vi "sub_GSlam_fill-Hnb.vi"(9 "edge in":T2, 10 "b":T1, 11 "H":T1 caption="H in") -> (2 "b out":T1 caption="b", 3 "H out":T1)   [LabVIEW 2019]
uses:
  <vilib>/Analysis/Matrix/Datatypes/RealMatrix.ctl
  Ctrl/cmd_common.ctl
  <vilib>/Analysis/Matrix/Numeric/Multiply/Multiply - RM,RM.vi
  <vilib>/Analysis/Matrix/Numeric/Add/Add - RM,RM.vi
  <vilib>/Analysis/Matrix/NI_Matrix.lvlib
panel:
  out "H matrix":dbl[][](graph)
  out "열의 개수":i32
  out "행의 개수":i32
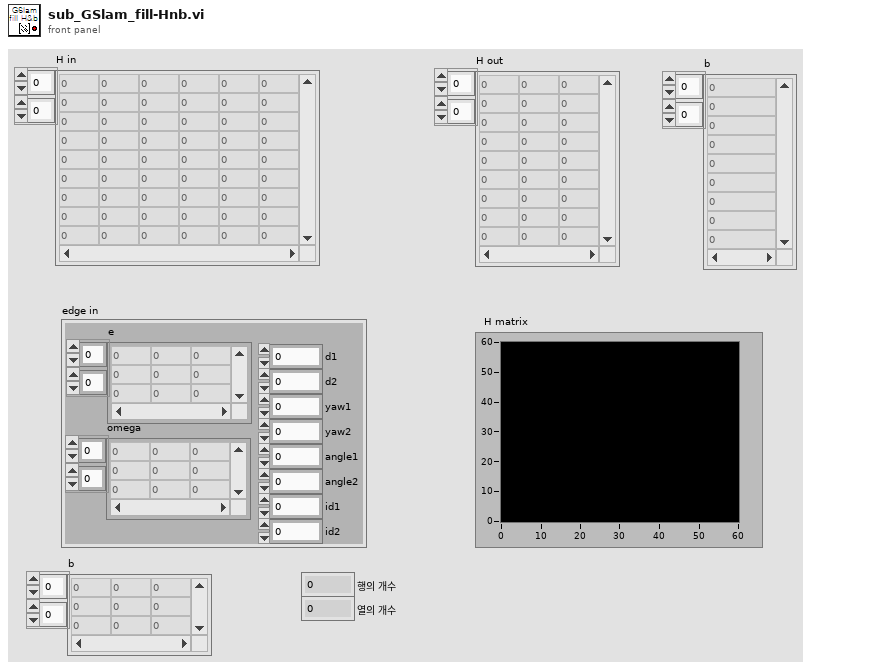
[diagram p1: front panel]
types:
  T1 = typedef "NI_Matrix.lvlib/RealMatrix.ctl" = dbl[][]
  T2 = cluster{"e":T1, "omega":T1, "d1":dbl, "d2":dbl, "yaw1":dbl, "yaw2":dbl, "angle1":dbl, "angle2":dbl, "id1":i32, "id2":i32}
  T3 = typedef "cmd_common.ctl" = enum16{"read", "write"}
  T4 = cluster{"Q Sim":T1, "R Sim":T1, "DT":dbl, "SIM_TIME":dbl, "MAX_RANGE":dbl, "STATE_SIZE":i32, "C_SIGMA 1":dbl, "C_SIGMA 2":dbl, "C_SIGMA 3":dbl, "MAX_ITR":u32}
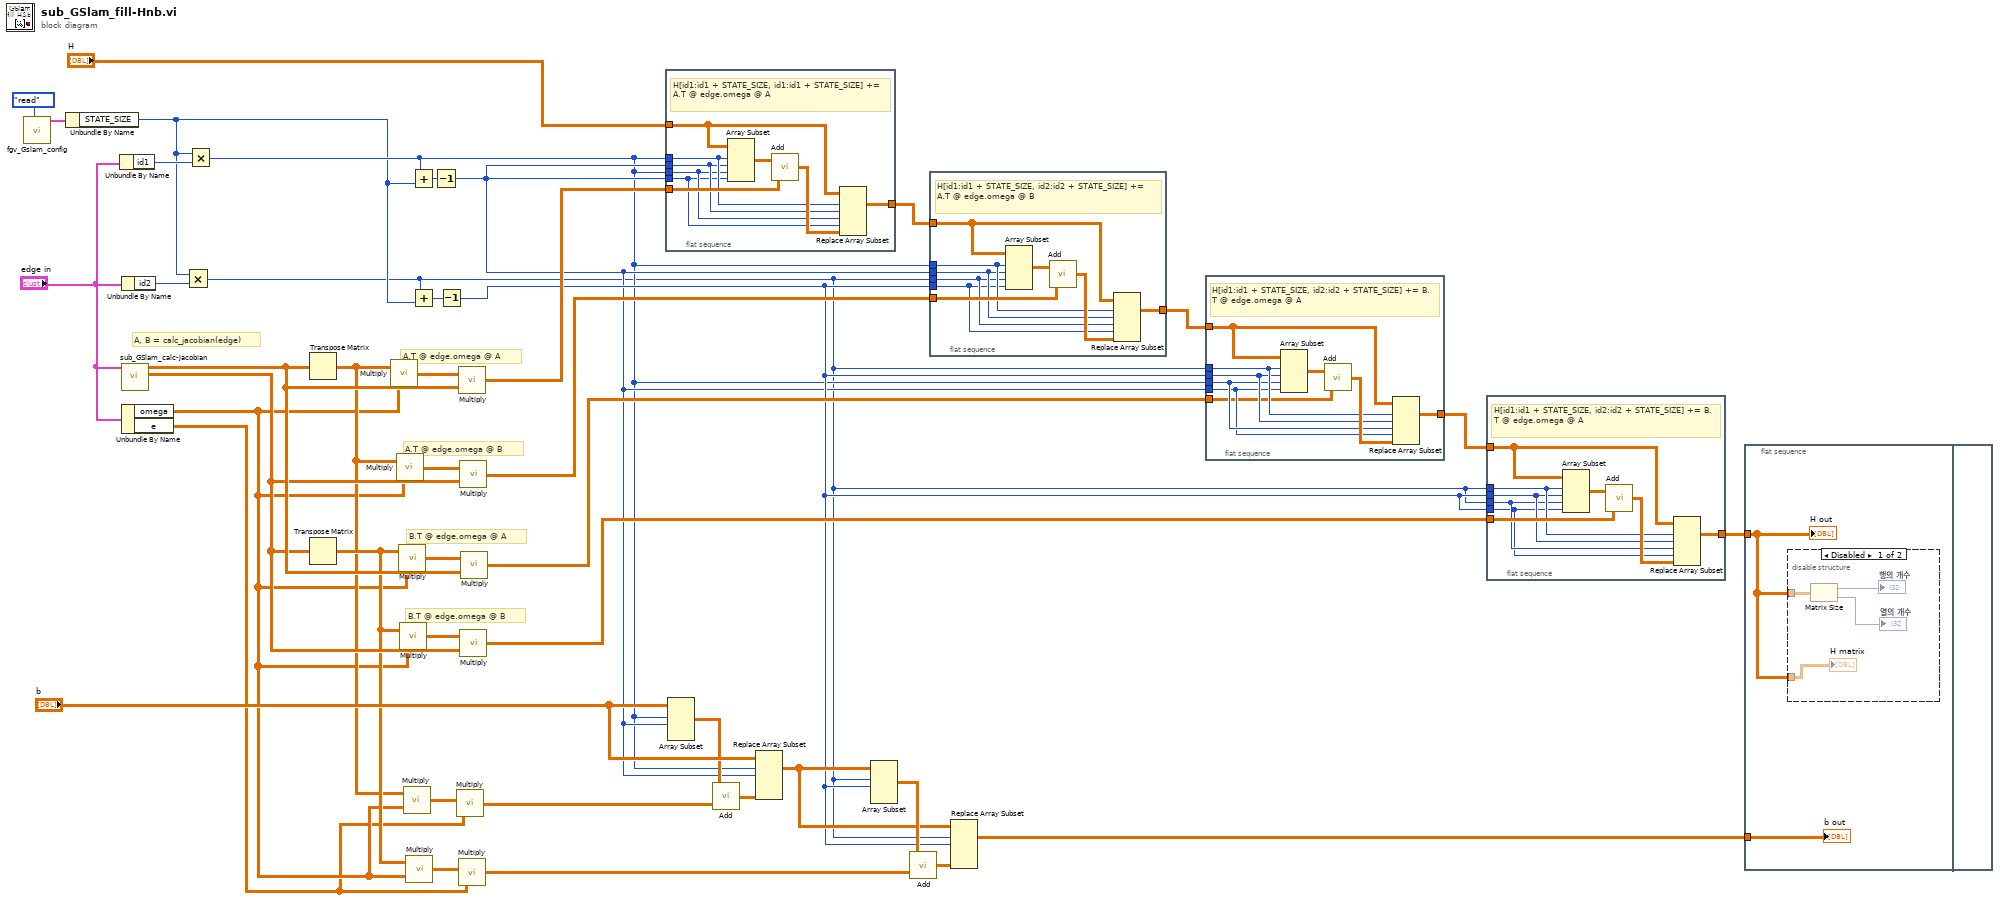
[diagram p0: block diagram]
diagram:
  # "B.T @ edge.omega @ B"
  # "B.T @ edge.omega @ A"
  # "A.T @ edge.omega @ B"
  # "A, B = calc_jacobian(edge)"
  # "A.T @ edge.omega @ A"
  n1 = call "fgv_Gslam_config.vi"("cmd"=cmd_common."read") -> ("G cofnig out"=w41:T4)  [unwired: 10 in]
  n2 = Unbundle By Name(w41) -> ("STATE_SIZE"=w6:i32)
  n3 = Unbundle By Name("edge in") -> ("id1"=w9:i32)
  n4 = Unbundle By Name("edge in") -> ("id2"=w7:i32)
  n5 = call "sub_GSlam_calc-jacobian.vi"("edge"="edge in") -> ("B"=w32:T1, "A"=w33:T1)  [unwired: 9 in]
  n6 = Unbundle By Name("edge in") -> ("omega"=w3:T1, "e"=w2:T1)
  n7 = Multiply(x=w6, y=w7) -> (x*y=w5:i32)
  n8 = Multiply(x=w6, y=w9) -> (x*y=w8:i32)
  n9 = Transpose Matrix(1:w33) -> (0:w4:T1)
  n10 = Transpose Matrix(1:w32) -> (0:w18:T1)
  n11 = call-poly <vilib>:"Multiply.vi"("Real Matrix B"=w3, "Real Matrix A"=w4) -> ("A * B"=w40:T1)
  n12 = call-poly <vilib>:"Multiply.vi"("Real Matrix B"=w3, "Real Matrix A"=w4) -> ("A * B"=w37:T1)
  n13 = call-poly <vilib>:"Multiply.vi"("Real Matrix B"=w3, "Real Matrix A"=w18) -> ("A * B"=w35:T1)
  n14 = call-poly <vilib>:"Multiply.vi"("Real Matrix B"=w3, "Real Matrix A"=w18) -> ("A * B"=w34:T1)
  n15 = call-poly <vilib>:"Multiply.vi"("Real Matrix B"=w3, "Real Matrix A"=w4) -> ("A * B"=w26:T1)
  n16 = call-poly <vilib>:"Multiply.vi"("Real Matrix B"=w3, "Real Matrix A"=w18) -> ("A * B"=w19:T1)
  n17 = Add(x=w8, y=w6) -> (x+y=w24:i32)
  n18 = Add(x=w5, y=w6) -> (x+y=w15:i32)
  n19 = Decrement(x=w24) -> (x-1=w10:i32)
  n20 = Decrement(x=w15) -> (x-1=w13:i32)
  n21 = call-poly <vilib>:"Multiply.vi"("Real Matrix B"=w2, "Real Matrix A"=w26) -> ("A * B"=w1:T1)
  n22 = call-poly <vilib>:"Multiply.vi"("Real Matrix B"=w33, "Real Matrix A"=w40) -> ("A * B"=w38:T1)
  n23 = call-poly <vilib>:"Multiply.vi"("Real Matrix B"=w2, "Real Matrix A"=w19) -> ("A * B"=w17:T1)
  n24 = call-poly <vilib>:"Multiply.vi"("Real Matrix B"=w32, "Real Matrix A"=w37) -> ("A * B"=w36:T1)
  n25 = call-poly <vilib>:"Multiply.vi"("Real Matrix B"=w32, "Real Matrix A"=w34) -> ("A * B"=w27:T1)
  n26 = call-poly <vilib>:"Multiply.vi"("Real Matrix B"=w33, "Real Matrix A"=w35) -> ("A * B"=w29:T1)
  n27 = flat-sequence {
    tunnel: w38 -> [w50]
    tunnel: "H" -> [w49]
    tunnel: w8 -> [w44]
    tunnel: w10 -> [w43]
    tunnel: [w47] -> w31
    tunnel: w8 -> [w46]
    tunnel: w10 -> [w45]
    frame #0 {
      # "H[id1:id1 + STATE_SIZE, id1:id1 + STATE_SIZE] += A.T @ edge.omega @ A"
      n28 = Array Subset(array=w49, index (row)=w46, length (row)=w45, index (col)=w44, length (col)=w43) -> (w51:T1)
      n29 = call-poly <vilib>:"Add.vi"("Real Matrix B"=w50, "Real Matrix A"=w51) -> ("A + B"=w48:T1)
      n30 = Replace Array Subset(array=w49, new element=w48, index (dim 0)=w46, index (dim 1)=w45, index (dim 2)=w44, index (dim 3)=w43) -> (w47:T1)
    }
  }
  n31 = Array Subset(array="b", index (row)=w8, length (row)=w10) -> (w23:T1)  [unwired: 2 in]
  n32 = call-poly <vilib>:"Add.vi"("Real Matrix B"=w1, "Real Matrix A"=w23) -> ("A + B"=w22:T1)
  n33 = Replace Array Subset(array="b", new element=w22, index (dim 0)=w8, index (dim 1)=w10) -> (w16:T1)  [unwired: 2 in]
  n34 = Array Subset(array=w16, index (row)=w5, length (row)=w13) -> (w20:T1)  [unwired: 2 in]
  n35 = call-poly <vilib>:"Add.vi"("Real Matrix B"=w17, "Real Matrix A"=w20) -> ("A + B"=w21:T1)
  n36 = flat-sequence {
    tunnel: w36 -> [w59]
    tunnel: w5 -> [w53]
    tunnel: w13 -> [w52]
    tunnel: w8 -> [w55]
    tunnel: w10 -> [w54]
    tunnel: [w58] -> w30
    tunnel: w31 -> [w56]
    frame #0 {
      # "H[id1:id1 + STATE_SIZE, id2:id2 + STATE_SIZE] += A.T @ edge.omega @ B"
      n37 = Array Subset(array=w56, index (row)=w55, length (row)=w54, index (col)=w53, length (col)=w52) -> (w60:T1)
      n38 = call-poly <vilib>:"Add.vi"("Real Matrix B"=w59, "Real Matrix A"=w60) -> ("A + B"=w57:T1)
      n39 = Replace Array Subset(array=w56, new element=w57, index (dim 0)=w55, index (dim 1)=w54, index (dim 2)=w53, index (dim 3)=w52) -> (w58:T1)
    }
  }
  n40 = Replace Array Subset(array=w16, new element=w21, index (dim 0)=w5, index (dim 1)=w13) -> (w14:T1)  [unwired: 2 in]
  n41 = flat-sequence {
    tunnel: w29 -> [w61]
    tunnel: [w63] -> _
    tunnel: w10 -> [w62]
    tunnel: w5 -> [w65]
    tunnel: w13 -> [w64]
    tunnel: [w68] -> w28
    tunnel: w30 -> [w66]
    tunnel: w8 -> [w63]
    frame #0 {
      # "H[id1:id1 + STATE_SIZE, id2:id2 + STATE_SIZE] += B.T @ edge.omega @ A"
      n42 = Array Subset(array=w66, index (row)=w65, length (row)=w64, index (col)=w63, length (col)=w62) -> (w69:T1)
      n43 = call-poly <vilib>:"Add.vi"("Real Matrix B"=w61, "Real Matrix A"=w69) -> ("A + B"=w67:T1)
      n44 = Replace Array Subset(array=w66, new element=w67, index (dim 0)=w65, index (dim 1)=w64, index (dim 2)=w63, index (dim 3)=w62) -> (w68:T1)
    }
  }
  n45 = flat-sequence {
    tunnel: w27 -> [w77]
    tunnel: w5 -> [w71]
    tunnel: w13 -> [w70]
    tunnel: w5 -> [w73]
    tunnel: w13 -> [w72]
    tunnel: [w76] -> w12
    tunnel: w28 -> [w74]
    tunnel: [w71] -> _
    frame #0 {
      # "H[id1:id1 + STATE_SIZE, id2:id2 + STATE_SIZE] += B.T @ edge.omega @ A"
      n46 = Array Subset(array=w74, index (row)=w73, length (row)=w72, index (col)=w71, length (col)=w70) -> (w78:T1)
      n47 = call-poly <vilib>:"Add.vi"("Real Matrix B"=w77, "Real Matrix A"=w78) -> ("A + B"=w75:T1)
      n48 = Replace Array Subset(array=w74, new element=w75, index (dim 0)=w73, index (dim 1)=w72, index (dim 2)=w71, index (dim 3)=w70) -> (w76:T1)
    }
  }
  n49 = flat-sequence {
    tunnel: w14 -> [w80]
    tunnel: w12 -> [w79]
    frame #0 {
      n50 = disable-structure shown="Disabled" {
        disable-tunnel: w79 -> [w84 _]
        disable-tunnel: w79 -> [w81 _]
        frame Disabled {
          n51 = Matrix Size(0:w84) -> (1:→"행의 개수":i32, 2:→"열의 개수":i32)
          "H matrix" <- w81
        }
        frame Enabled {
        }
      }
      "H out" <- w79
      "b out" <- w80
    }
    frame #1 {
    }
  }
